vi "ResizeSubpaneltoPane.vi"(5 "Borders in Percent(T) or Pixels (F)":bool, 6 "Adjust":u16(ring) items=["Height", "Width", "Both"], 7 "Minimal":T1, 8 "error in (no error)":errorcluster, 9 "Borders":T2, 10 "SubPanel":refnum<vi>, 11 "PentaPanesGUI in":refnum<class "PentaPanes.lvclass">) -> (0 "error out":errorcluster, 3 "PentaPanesGUI out":refnum<class "PentaPanes.lvclass">)   [LabVIEW 2022 SP3, in "PentaPanesLibrary.lvlib" / "PentaPanes.lvclass"]
uses:
  PentaPanes.lvclass
  BordersCluster.ctl
  <vilib>/Utility/miscctls.llb/LVBoundsTypeDef.ctl
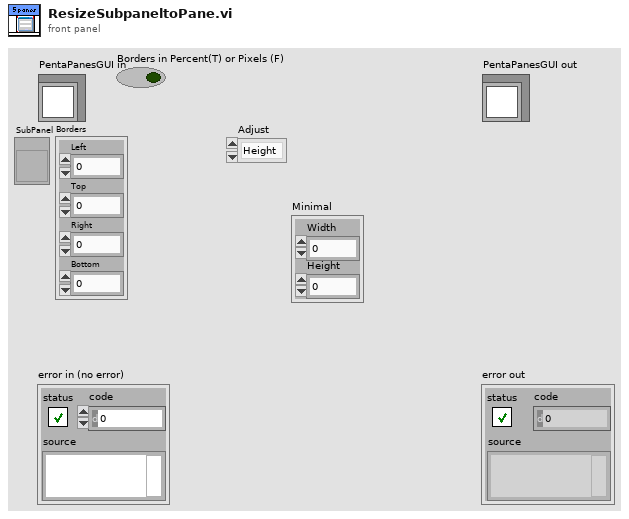
[diagram p1: front panel]
types:
  T1 = typedef "LVBoundsTypeDef.ctl" = cluster{"Width":i32, "Height":i32}
  T2 = typedef "PentaPanesLibrary.lvlib/PentaPanes.lvclass/BordersCluster.ctl" = cluster{"Left":i32, "Top":i32, "Right":i32, "Bottom":i32}
  T3 = typedef "LVBoundsTypeDef.ctl" = cluster{"Width":u32, "Height":u32}
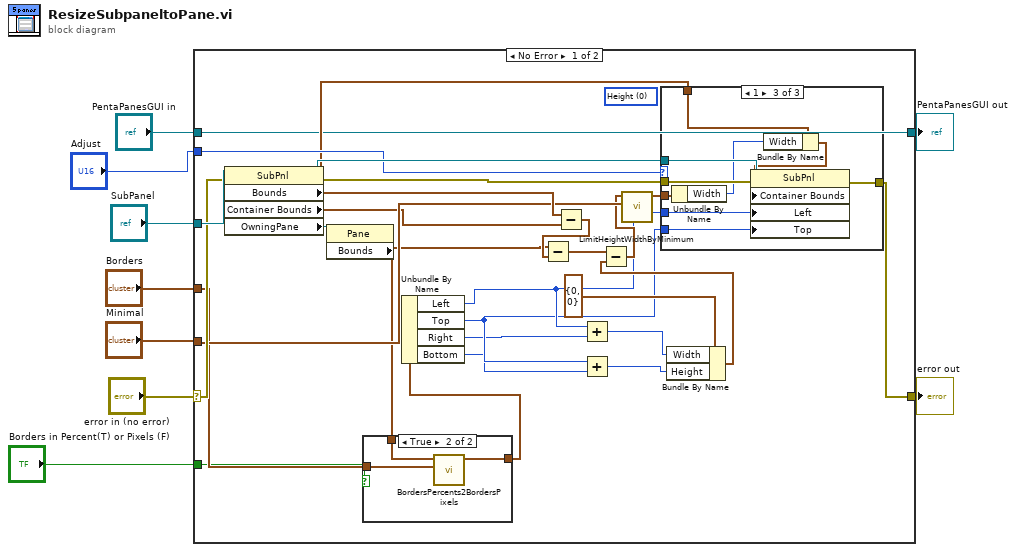
[diagram p0: block diagram]
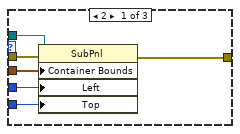
[diagram p3: hidden frame]
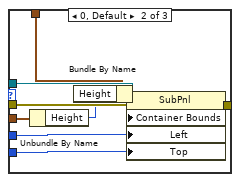
[diagram p4: hidden frame]
diagram:
  n1 = case shown="No Error" "error in (no error)" {
    selector: "error in (no error)" -> [w31 w66]
    tunnel: [w24 w66] -> w8
    tunnel: [w10 w65] -> w6
    tunnel: "PentaPanesGUI in" -> [w10 w65]
    tunnel: "SubPanel" -> [w32 _]
    tunnel: "Borders" -> [w14 _]
    tunnel: "Adjust" -> [w23 _]
    tunnel: "Minimal" -> [w21 _]
    tunnel: "Borders in Percent(T) or Pixels (F)" -> [w12 _]
    frame No Error {
      (unwired) u16 0 items=["Height", "Width", "Both"] ("Adjust")
      n2 = property class="SubPnl"(reference=w32, error in=w31) -> (reference out=w33:refnum<vi>, error out=w25:errorcluster, "Bounds"=w36:T3, "Container Bounds"=w11:T3, "OwningPane"=w34:refnum<vi>)
      n3 = property class="Pane"(reference=w34) -> ("Bounds"=w17:T3)  [unwired: 1 in, 2 out]
      n4 = case shown="True" w12 {
        tunnel: w17 -> [_ w40]
        tunnel: w14 -> [w37 w39]
        tunnel: [w37 w38] -> w13
        frame False {
        }
        frame True {
          n5 = call "BordersPercents2BordersPixels.vi"("Borders in"=w39, "Bounds"=w40) -> ("Borders out"=w38:T2)  [unwired: 9 in]
        }
      }
      n6 = Unbundle By Name(w13) -> ("Left"=w19:i32, "Top"=w18:i32, "Right"=w16:i32, "Bottom"=w15:i32)
      n7 = Subtract(x=w36, y=w11) -> (x-y=w35:T3)
      n8 = Subtract(x=w17, y=w35) -> (x-y=w27:T3)
      n9 = Add(x=w19, y=w16) -> (x+y=w29:i32)
      n10 = Add(x=w18, y=w15) -> (x+y=w28:i32)
      n11 = Bundle By Name(cluster=T1 {"Width"=0, "Height"=0} ("x-y"), "Width"=w29, "Height"=w28) -> (w26:T1)
      n12 = Subtract(x=w27, y=w26) -> (x-y=w20:T3)
      n13 = call "LimitHeightWidthByMinimum.vi"("Minimal"=w21, "Height Width in"=w20) -> ("Limited Height Width out"=w22:T1)  [unwired: 9 in]
      n14 = case shown="1" w23 {
        tunnel: w33 -> [w46 w55 w64]
        tunnel: w22 -> [w45 w50 w59]
        tunnel: w19 -> [w44 w54 w63]
        tunnel: w18 -> [w43 w53 w62]
        tunnel: w25 -> [w42 w52 w61]
        tunnel: [w41 w51 w60] -> w24
        tunnel: w11 -> [_ w48 w58]
        frame 2 {
          n15 = property class="SubPnl"(reference=w46, error in=w42, "Container Bounds"=w45, "Left"=w44, "Top"=w43) -> (error out=w41:errorcluster)  [unwired: 1 out]
        }
        frame 0, Default {
          n16 = Unbundle By Name(w50) -> ("Height"=w47:i32)
          n17 = Bundle By Name(cluster=w48, "Height"=w47) -> (w49:T3)
          n18 = property class="SubPnl"(reference=w55, error in=w52, "Container Bounds"=w49, "Left"=w54, "Top"=w53) -> (error out=w51:errorcluster)  [unwired: 1 out]
        }
        frame 1 {
          n19 = Unbundle By Name(w59) -> ("Width"=w57:i32)
          n20 = Bundle By Name(cluster=w58, "Width"=w57) -> (w56:T3)
          n21 = property class="SubPnl"(reference=w64, error in=w61, "Container Bounds"=w56, "Left"=w63, "Top"=w62) -> (error out=w60:errorcluster)  [unwired: 1 out]
        }
      }
    }
    frame Error {
    }
  }
  "error out" <- w8
  "PentaPanesGUI out" <- w6
